vi "GT Link Capture Offset.vi"(8 "error in (no error)":errorcluster caption="错误输入（无错误）", 9 "source":i16, 10 "encoder":i16, 11 "cardNum":i16) -> (0 "error out":errorcluster caption="错误输出", 3 "function return":i16)   [LabVIEW 2020, in "gts1.lvlib"]
doc: "GT_API GT_LinkCaptureOffset(short cardNum,short encoder,short source);"
uses:
  gts1.lvlib
  dll/32bit/multi_card/gts.dll
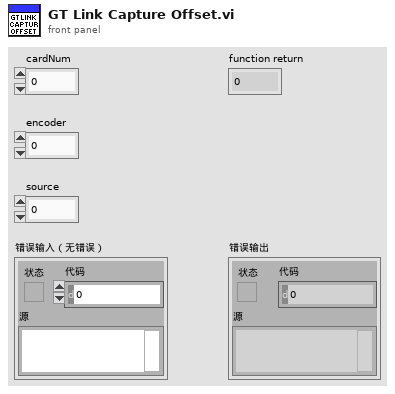
[diagram p1: front panel]
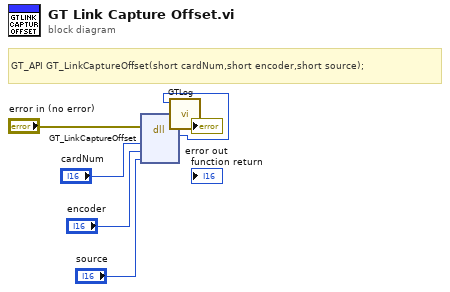
[diagram p0: block diagram]
diagram:
  # "GT_API GT_LinkCaptureOffset(short cardNum,short encoder,short source);"
  n1 = dll-call lib="C:/1228/dll/32bit/multi_card/gts.dll" fn="GT_LinkCaptureOffset"(error in="error in (no error)", "cardNum"="cardNum", "encoder"="encoder", "source"="source") -> (error out=w3:errorcluster, w1:i16)  [unwired: 5 in, 1 out]
  n2 = call "GTLog.vi"("error in (no error)"=w3, "Numeric"=w1) -> ("error out"=→"error out":errorcluster)  [unwired: 9 in]
